vi "运维调试_氨氮.vi"() -> ()   [LabVIEW 2016, in "斯坦道氨氮.lvlib"]
uses:
  <vilib>/Utility/miscctls.llb/LVPointTypeDef.ctl
  <vilib>/Utility/config.llb/NI_LVConfig.lvlib
  <vilib>/ptbypt/NI_PtbyPt.lvlib
panel:
  out "固件版本号":string
  in  "定时设置":cluster{"启动":bool, "控制命令":T1, "测量参数":T2}(xcontrol)
  out "模块版本号":string
  in  "校准按钮":T3
  out "单位:":T4(ring)
  out "运行状态":T5 {"数据时间:" format="%<%y/%m/%d %H:%M:%S>T"; "仪器时间:" format="%<%y/%m/%d %H:%M:%S>T"}
  out "二级权限":bool
  out "一级权限":bool
  out "输入密码":u32
  out "布尔":bool
  in  "仪器参数设置":bool
  in  "流程固件":bool
  in  "量程参数读取":T6
  in  "模块启用":bool
  in  "串口设置":bool
  in  "公式一键写入":bool
  in  "流程路径":path=path "C:/Users/STD/Documents/斯坦道流程文件/流程.xml"
  in  "曲线模型":cluster{"X^2":dbl, "X":dbl, "B":dbl, "r^2":dbl}(xcontrol)
  out "字符串":string
  in  "质控参数设置":bool
  in  "自动测试量程配置":T7
  out "温度2":sgl
  out "温度1":sgl
  out "ADC":sgl
  in  "数组":string[](array[string])
  in  "量程切换阈值写入":bool
  in  "量程切换阈值读取":bool
  in  "参数下拉列表":enum16{"总磷", "总氮", "氨氮"}(ring)=enum."氨氮"
  in  "量程下拉列表":enum16{"低量程", "高量程"}(ring)
  in  "测量模式下拉列表":enum16{"水样测量", "零点核查", "跨度核查", "标样核查", "加标回收"}(ring)
  in  "公式":cluster{"X^2":dbl, "X":dbl, "b":dbl}
  in  "写公式":bool
  in  "读公式":bool
  in  "返回":bool
  in  "设置":bool
  out "集成报警信息":string
  in  "停止":bool
  in  "手动启动":bool
  in  "单步测试":bool
  out "F3":sgl format="%#.6f"
  out "F2":sgl format="%#.6f"
  out "F1":sgl format="%#.6f"
  out "F0":sgl format="%#.6f"
  out "多列列表框":i32(listbox)
  # "参数设置"
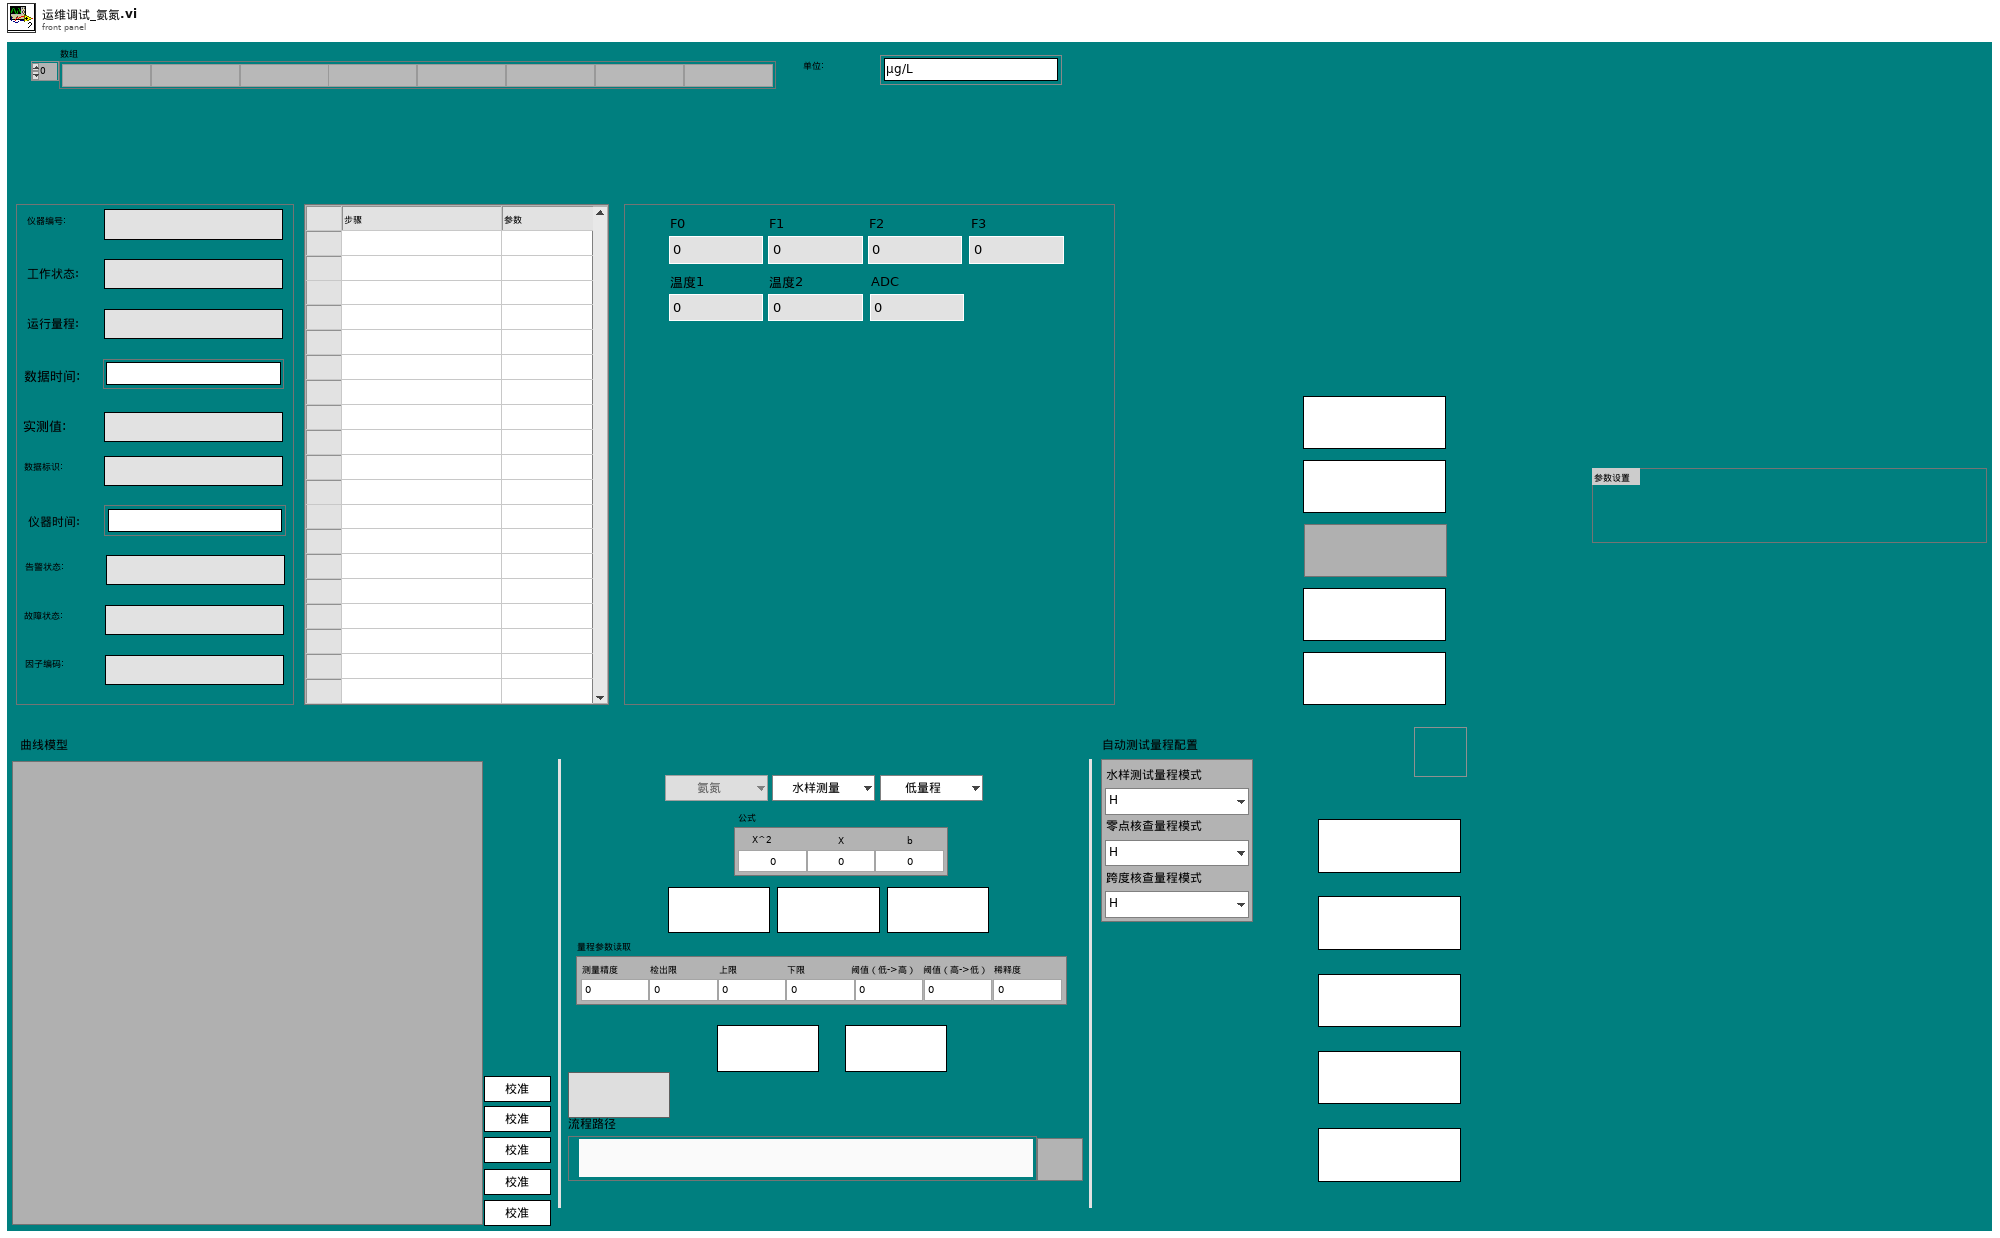
[diagram p1: front panel]
types:
  T1 = typedef "定时设置.xctl/国标控制命令.ctl" = enum16{"启动测量", "标样核查", "零点核查", "跨度核查", "空白测试", "平行样测试", "加标回收", "空白校准", "标样校准", "初始化（清洗）", "停止测试", "仪器重启", "校时", "模式设置", "测量间隔设置"}
  T2 = typedef "定时设置.xctl/测量参数.ctl" = u16
  T3 = cluster{"校准1":bool, "校准2":bool, "校准3":bool, "校准4":bool, "校准5":bool}
  T4 = enum16{"μg/L", "mg/L", "ppm", "mg/m3", "cm", "ppb", "μg/m3", "%", "nmol/mol", "μmol/mol", "MPN/L", "MPN/100ml", "ng/m3", "NTU", "无量纲", "mS/cm", "μS/cm", "℃", "mV", "cells/mL"}
  T5 = cluster{"仪器编号:":string, "工作状态:":string, "运行量程: ":string, "数据时间:":timestamp, "实测值:":string, "数据标识: ":string, "仪器时间:":timestamp, "告警状态: ":string, "故障状态:  ":string, "因子编码:":string}
  T6 = cluster{"测量精度":dbl, "检出限":dbl, "上限":dbl, "下限":dbl, "阈值（低->高）":dbl, "阈值（高->低）":dbl, "稀释度":dbl}
  T7 = cluster{"水样测试量程模式":enum16{"H", "L", "AUTO"}, "空白核查量程模式":enum16{"H", "L", "AUTO"}, "跨度核查量程模式":enum16{"H", "L", "AUTO"}}
  T8 = cluster{"时间源选择":enum16{"系统时间源", "仪器时间源"}, "外部时间源":timestamp}
  T9 = enum16{"空闲", "水样测试", "标样核查", "零点核查", "跨度核查", "空白测试", "平行样测试", "加标回收", "空白校准", "标样校准", "初始化（清洗）"}
  T10 = cluster{"系统时间":timestamp, "工作状态":enum16{"空闲", "水样测试", "标样核查", "零点核查", "跨度核查", "空白测试", "平行样测试", "加标回收", "空白校准", "标样校准", "初始化（清洗）"}, "测量模式":enum16{"待机", "连续模式", "周期模式", "定点模式", "受控模式", "手动模式"}, "告警代码":u16, "故障代码":u16, "日志代码":u16, "软件版本":u16, "F0":sgl, "F1":sgl, "F2":sgl, "F3":sgl, "T":sgl, "H":sgl, "id":u16, "flowid":u16, "量程":u16, "总磷控温温度1":sgl, "营养盐控温温度2":sgl, "ADC":sgl}
  T11 = enum32{"Bad", "Idle", "Run top level", "Running"}
  T12 = typedef "定时设置.xctl/周期模式设置.ctl" = enum16{"不启用", "定点模式", "间隔模式"}
  T13 = typedef "定时设置.xctl/定点周期设置.ctl" = cluster{"启动命令":T14, "启动命令 2":T14, "启动命令 3":T14, "启动命令 4":T14, "启动命令 5":T14, "启动命令 6":T14, "启动命令 7":T14, "启动命令 8":T14, "启动命令 9":T14, "启动命令 10":T14, "启动命令 11":T14, "启动命令 12":T14, "启动命令 13":T14, "启动命令 14":T14, "启动命令 15":T14, "启动命令 16":T14, "启动命令 17":T14, "启动命令 18":T14, "启动命令 19":T14, "启动命令 20":T14, "启动命令 21":T14, "启动命令 22":T14, "启动命令 23":T14, "启动命令 24":T14}
  T14 = typedef "定时设置.xctl/启动命令选择.ctl" = u16
  T15 = typedef "定时设置.xctl/间隔启动设置.ctl" = cluster{"启动命令":T14, "启动间隔":dbl, "启动次数":i32}
  T16 = cluster{"周期模式":T12, "定点周期":T13, "间隔启动":T15, "启动参数":u16}
  T17 = cluster{"周期模式":T12, "定点周期":T13, "间隔启动":T15, "测量参数":T2}
  T18 = typedef "LVPointTypeDef.ctl" = cluster{"Horizontal":i16, "Vertical":i16}
  T19 = cluster{"因子编码":u32, "单位":u16, "标样参考值":sgl, "水样数据时间":timestamp, "水样实测值":sgl, "水样数据标识":string, "标样数据时间":timestamp, "标样实测值":sgl, "标样数据标识":string, "空白数据时间":timestamp, "空白实测值":sgl, "空白数据标识":string, "零点核查数据时间":timestamp, "零点核查实测值":sgl, "零点核查数据标识":string, "跨度核查数据时间":timestamp, "跨度核查实测值":sgl, "跨度核查数据标识":string, "加标回收数据时间":timestamp, "加标回收实测值":sgl, "加标回收数据标识":string, "平行样数据时间":timestamp, "平行样实测值":sgl, "平行样数据标识":string, "F0":sgl, "F1":sgl, "F2":sgl, "F3":sgl, "F4":sgl, "F5":sgl, "F6":sgl, "F7":sgl, "温度":sgl, "湿度":sgl, "X值":sgl, "fidrange":u16}
  T20 = cluster{"Major":u16, "Minor":u16, "Fix":u16, "Build":u16}
  T21 = typedef "NI_LVConfig.lvlib/Config Data RefNum.ctl" = refnum<k1>
  T22 = enum8{"Enabled", "Disabled", "Disabled and Grayed Out"}
  T23 = cluster{"时间标识":timestamp, "设备":string, "日志信息":string, "备注":string}
  T24 = cluster{"参数":string, "报警内容":string, "报警分析":string}
  T25 = cluster{"启动模式":enum16{"跨度核查", "水样测量", "空白核查", "标样核查", "加标回收"}, "启动参数":u16, "量程":enum16{"低量程", "高量程"}}
  T26 = cluster{"时间标识":timestamp, "设备":string, "日志信息":string, "流程参数":string}
  T27 = typedef "LVRowAndColumnUnsignedTypeDef.ctl" = cluster{"Row":u32, "Column":u32}
  T28 = cluster{"参数下拉列表":enum16{"总磷", "总氮", "氨氮"}, "测量模式下拉列表":enum16{"水样测量", "零点核查", "跨度核查", "标样核查", "加标回收"}, "量程下拉列表":enum16{"低量程", "高量程"}}
  T29 = cluster{"站号":u16, "量程切换":enum32{"H", "L", "AUTO"}, "控制命令":enum16{"启动测量", "标样核查", "零点核查", "跨度核查", "空白测试", "平行样测试", "加标回收", "空白校准", "标样校准", "初始化（清洗）", "停止测试", "仪器重启", "校时", "模式设置", "测量间隔设置"}, "模式设置":enum16{"待机", "连续模式", "周期模式", "定点模式", "受控模式", "手动模式"}, "测量间隔":u16}
  T30 = cluster{"标液浓度1":dbl, "标液浓度2":dbl, "标液浓度3":dbl, "标液浓度4":dbl, "标液浓度5":dbl}
  T31 = cluster{"跨度值":dbl, "零点标准液浓度":dbl, "跨度标准液浓度":dbl, "标准液标准浓度":dbl}
  T32 = cluster{"确定":bool, "跨度值":dbl, "零点标准液浓度":dbl, "跨度标准液浓度":dbl, "标准液标准浓度":dbl}
  T33 = cluster{"测量量程":dbl, "测量精度":dbl, "测量间隔":dbl, "消解温度":dbl, "消解时长":dbl, "空白校准时间":timestamp, "曲线截距":dbl, "曲线斜率":dbl, "测量检出限":dbl, "测量信号值":dbl, "线性相关系数":dbl, "二次多项式系数":dbl, "标样校准时间":timestamp, "稀释倍数":dbl, "三项式系数":dbl, "空白标定系数":dbl, "量程系数":dbl, "F0/ORPA":dbl, "F1/ORPB":dbl, "F2/ORPK":dbl, "F3":dbl, "F4":dbl, "F5":dbl, "F6":dbl, "F7":dbl, "X0/滴定数":dbl, "量程":dbl}
  T34 = cluster{"确定":bool, "测量量程":dbl, "测量精度":dbl, "测量间隔":dbl, "消解温度":dbl, "消解时长":dbl, "空白校准时间":timestamp, "曲线截距":dbl, "曲线斜率":dbl, "测量检出限":dbl, "测量信号值":dbl, "线性相关系数":dbl, "二次多项式系数":dbl, "标样校准时间":timestamp, "稀释倍数":dbl, "三项式系数":dbl, "空白标定系数":dbl, "量程系数":dbl, "F0/ORPA":dbl, "F1/ORPB":dbl, "F2/ORPK":dbl, "F3":dbl, "F4":dbl, "F5":dbl, "F6":dbl, "F7":dbl, "X0/滴定数":dbl, "量程":dbl}
  T35 = cluster{"测量精度":u16, "检出限":dbl, "上限":dbl, "下限":dbl, "阈值（低->高）":dbl, "阈值（高->低）":dbl, "稀释度":dbl}
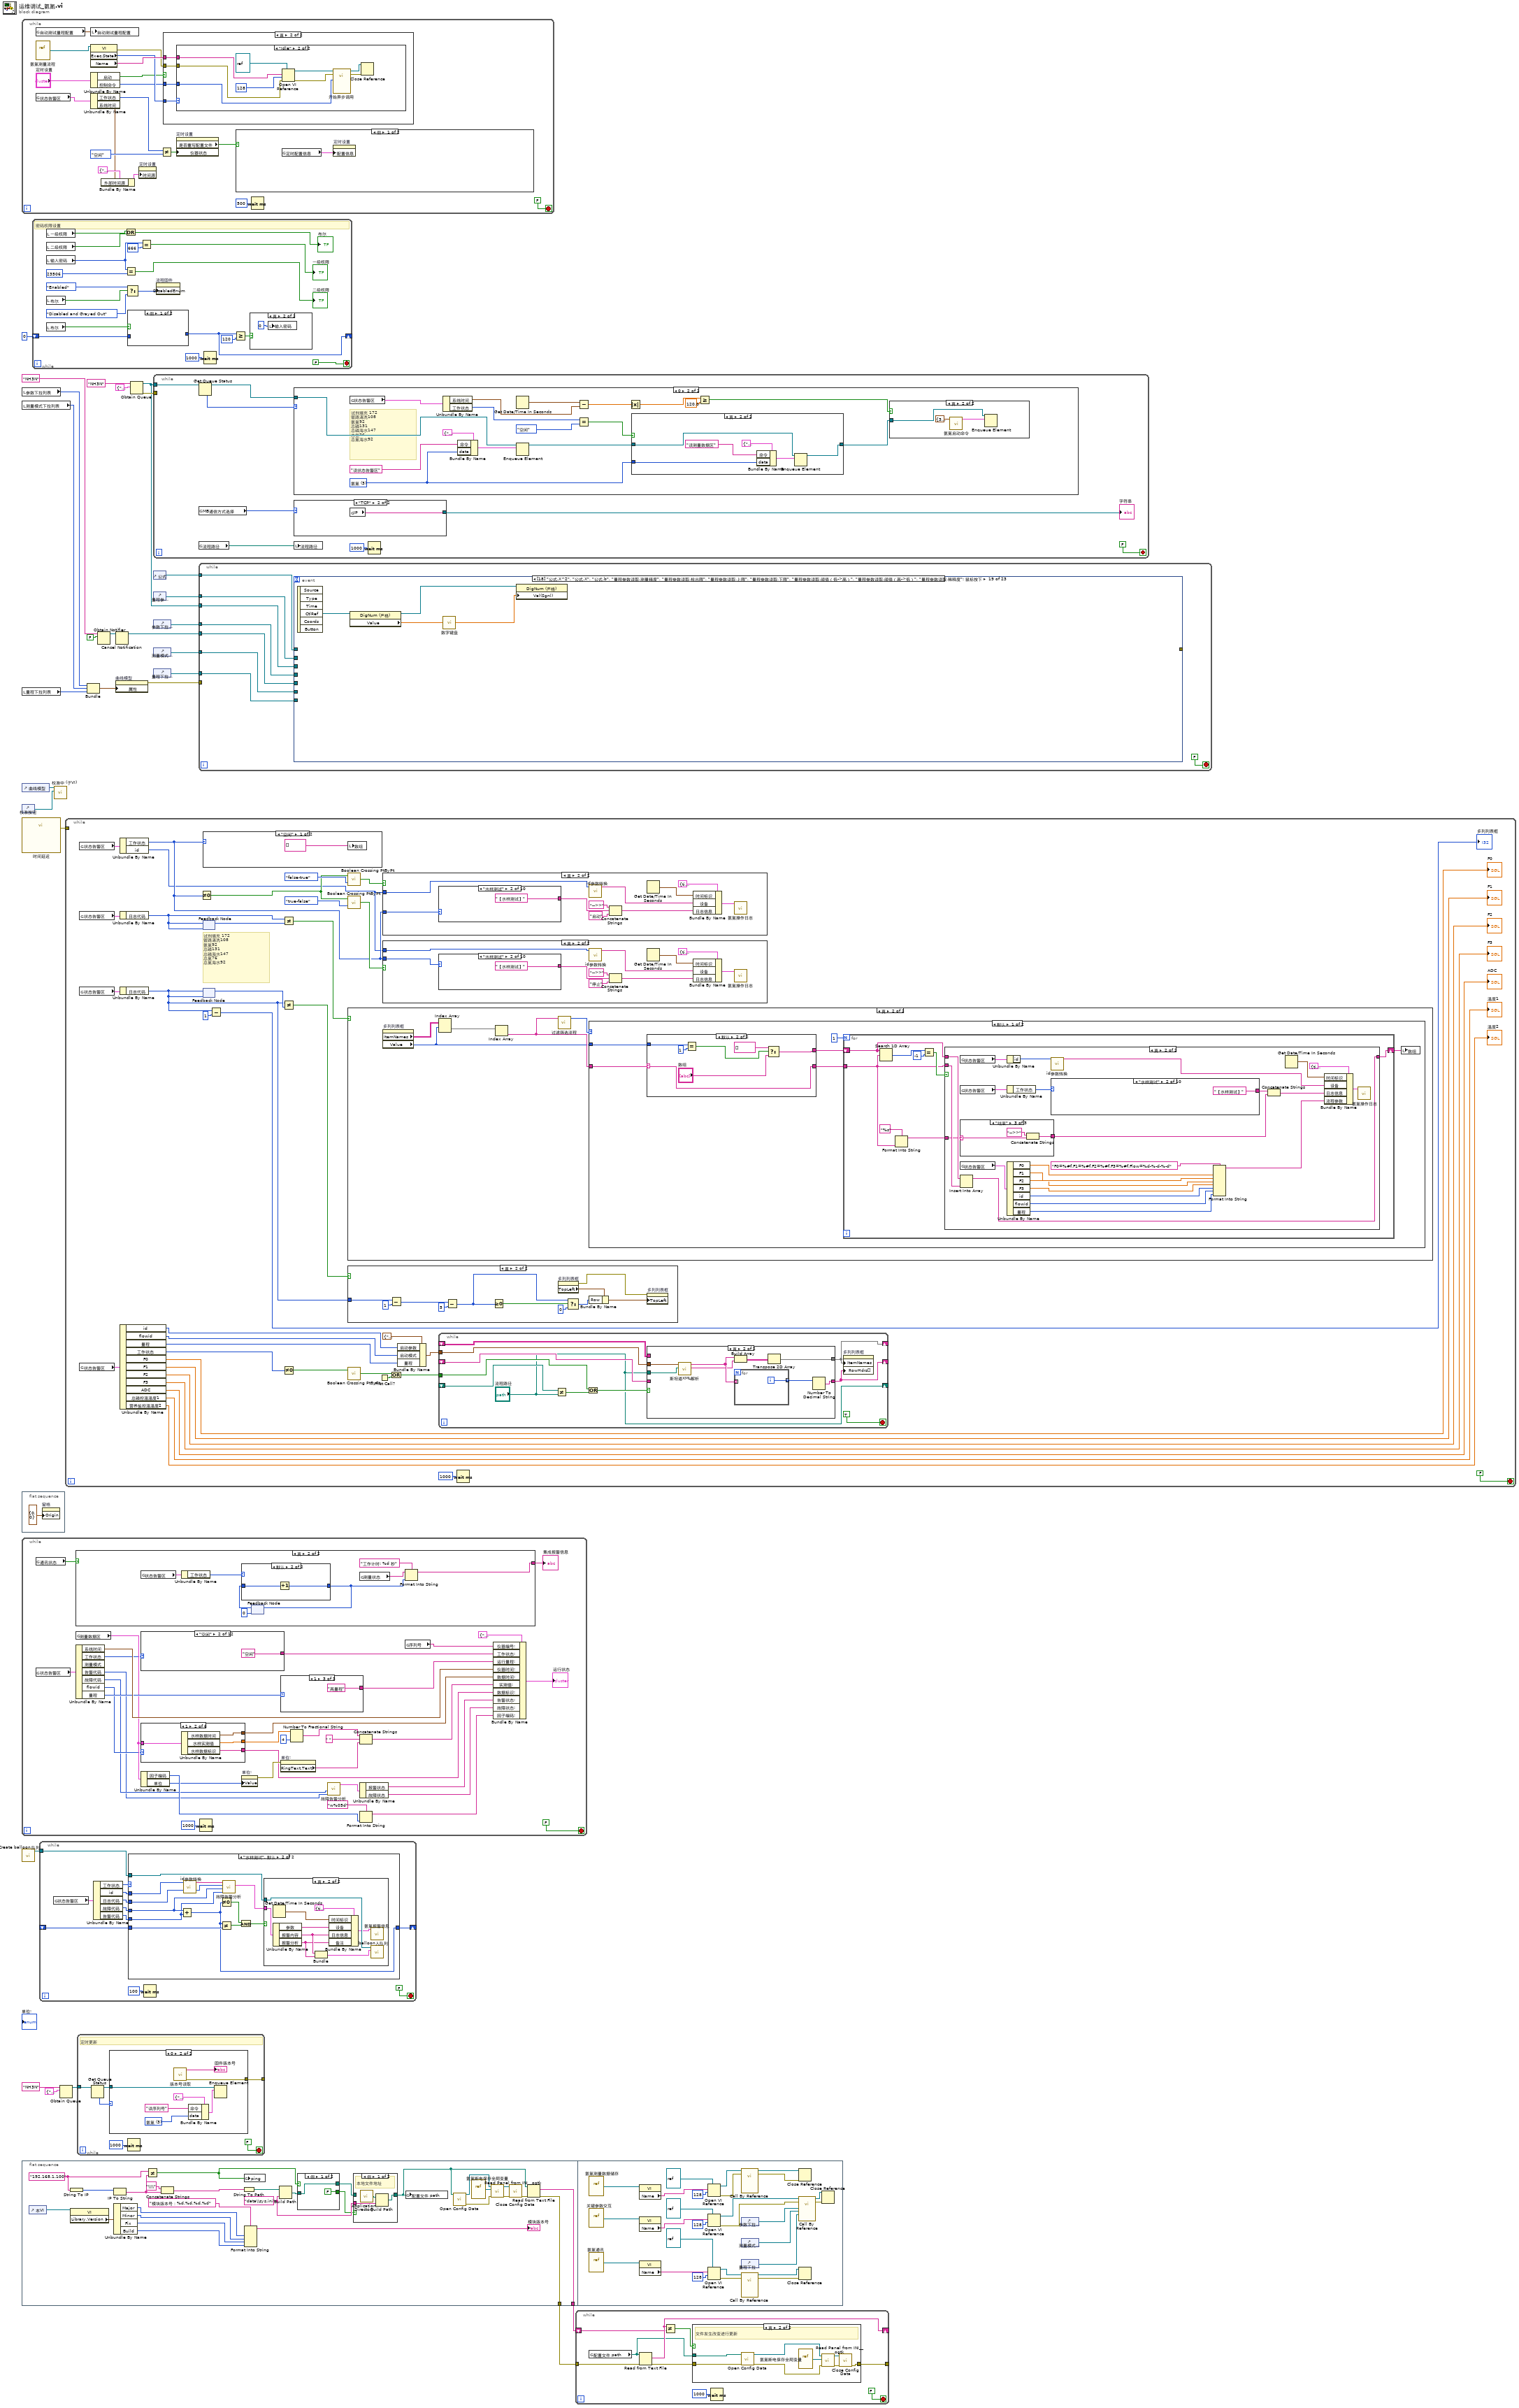
[diagram p0: block diagram]
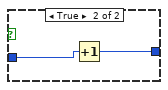
[diagram p6: hidden frame]
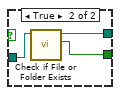
[diagram p7: hidden frame]
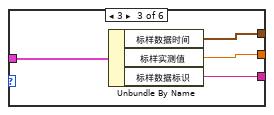
[diagram p11: hidden frame]
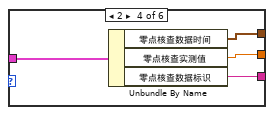
[diagram p12: hidden frame]
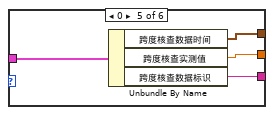
[diagram p13: hidden frame]
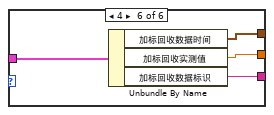
[diagram p14: hidden frame]
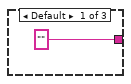
[diagram p15: hidden frame]
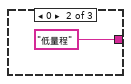
[diagram p16: hidden frame]
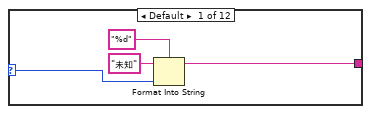
[diagram p17: hidden frame]
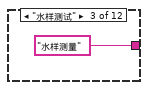
[diagram p18: hidden frame]
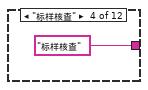
[diagram p19: hidden frame]
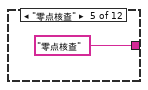
[diagram p20: hidden frame]
diagram:
  n1 = while {
    stop <- FALSE stop-if-true
    n2 = global read "氨氮断电保存全局变量.vi" "自动测试量程配置"() -> (w44:T7)
    n3 = vi-ref "氨氮测量流程.vi"() -> (w40:refnum<vi>)
    n4 = global read "VAR氨氮全局变量.vi" "状态告警区"() -> (w43:T10)
    n5 = local write "自动测试量程配置"(w44) -> ()
    n6 = property class="VI"(reference=w40) -> (error out=w37:errorcluster, "Exec.State"=w38:T11, "Name"=w39:string)  [unwired: 1 in, 1 out]
    n7 = Unbundle By Name("定时设置") -> ("启动"=w35:bool, "控制命令"=w34:T1)
    n8 = Unbundle By Name(w43) -> ("工作状态"=w42:T9, "系统时间"=w29:timestamp)
    n9 = Bundle By Name(cluster=T8 {"时间源选择"=enum."仪器时间源", "外部时间源"=timestamp(0 s since 1904-01-01)} ("时间源"), "外部时间源"=w29) -> (w30:T8)
    n10 = property on="定时设置" class="定时设置 (严格)"("时间源"=w30) -> ()  [unwired: 2 in, 2 out]
    n11 = Not Equal?(x=w42, y=T9."空闲") -> (x != y?=w32:bool)
    n12 = case shown="真" w35 {
      tunnel: w39 -> [_ w54]
      tunnel: w34 -> [_ w53]
      tunnel: w38 -> [_ w52]
      tunnel: w37 -> [_ w51]
      frame False {
      }
      frame True {
        n13 = case shown="\"Idle\"" w52 {
          tunnel: w54 -> [_ w59]
          tunnel: w53 -> [_ w57]
          tunnel: w51 -> [_ w55]
          frame "Bad", Default {
          }
          frame "Idle" {
            n14 = Open VI Reference(type specifier VI Refnum (for type only)=refnum<vi> refnum, vi path=w59, options=128 ("选项"), error in (no error)=w55) -> (vi reference=w60:refnum<vi>, error out=w61:errorcluster)  [unwired: 2 in]
            n15 = call-by-ref "开始异步调用"(reference=w60, error in=w61, "控制命令"=w57) -> (reference out=w62:refnum<vi>, error out=w63:errorcluster)  [unwired: 11 in]
            n16 = Close Reference(reference=w62, error in (no error)=w63) -> ()  [unwired: 1 out]
          }
        }
      }
    }
    n17 = property on="定时设置" class="定时设置 (严格)"("仪器状态"=w32) -> ("是否重写配置文件"=w33:bool)  [unwired: 2 in, 2 out]
    n18 = case shown="假" w33 {
      frame False {
        n19 = global read "氨氮断电保存全局变量.vi" "定时配置信息"() -> (w47:T16)
        n20 = property on="定时设置" class="定时设置 (严格)"("配置信息"=w47) -> ()  [unwired: 2 in, 2 out]
      }
      frame True {
        n21 = flat-sequence {
          tunnel: [w49] -> _
          frame #0 {
            n22 = property on="定时设置" class="定时设置 (严格)"() -> ("配置信息"=w48:T17)  [unwired: 2 in, 2 out]
            n23 = global write "氨氮断电保存全局变量.vi" "定时配置信息"(w48) -> ()
          }
          frame #1 {
            n24 = call "配置文件保存.vi"() -> ("错误输出"=w49:errorcluster)  [unwired: 11 in]
          }
          frame #2 {
            n25 = property on="定时设置" class="定时设置 (严格)"("是否重写配置文件"=FALSE) -> ()  [unwired: 2 in, 2 out]
          }
        }
      }
    }
    n26 = Wait (ms)(milliseconds to wait=u32 500 ("等待时间（毫秒）")) -> ()  [unwired: 1 out]
  }
  n27 = local read "参数下拉列表"() -> (w9:enum16{"总磷", "总氮", "氨氮"})
  n28 = local read "测量模式下拉列表"() -> (w8:enum16{"水样测量", "零点核查", "跨度核查", "标样核查", "加标回收"})
  n29 = local read "量程下拉列表"() -> (w7:enum16{"低量程", "高量程"})
  n30 = control-ref of="曲线模型"() -> (w3:refnum<vi>)
  n31 = control-ref of="校准按钮"() -> (w2:refnum<vi>)
  n32 = call "时间延迟"() -> ("error out"=w20:errorcluster)  [unwired: 11 in]
  n33 = flat-sequence {
    frame #0 {
      n34 = property on="窗格" class="Pane"("Origin"=T18 {"Horizontal"=0, "Vertical"=0} ("原点")) -> ()  [unwired: 2 in, 2 out]
    }
  }
  n35 = while {
    stop <- FALSE stop-if-true
    n36 = global read "VAR氨氮全局变量.vi" "通讯状态"() -> (w95:bool)
    n37 = global read "VAR氨氮全局变量.vi" "状态告警区"() -> (w93:T10)
    n38 = case shown="真" w95 {
      tunnel: ["通讯异常" ("集成报警信息") w138] -> w94
      frame False {
      }
      frame True {
        n39 = global read "VAR氨氮全局变量.vi" "状态告警区"() -> (w144:T10)
        n40 = Unbundle By Name(w144) -> ("工作状态"=w143:T9)
        n41 = feedback #1(0) -> (w141:i32)
        n42 = case shown="默认" w143 {
          tunnel: w141 -> [_ w146]
          tunnel: [_ w145] -> w139
          frame "空闲" {
          }
          frame Default {
            n43 = Increment(x=w146) -> (x+1=w145:i32)
          }
        }
        n44 = feedback-in #1(w139) -> ()
        n45 = global read "VAR氨氮全局变量.vi" "测量状态"() -> (w137:string)
        n46 = Format Into String(format string="工作计时: %d 秒" ("格式字符串"), initial string=w137, w139) -> (resulting string=w138:string)  [unwired: 1 in, 1 out]
      }
    }
    "集成报警信息" <- w94
    n47 = global read "VAR氨氮全局变量.vi" "测量数据区"() -> (w85:T19)
    n48 = Unbundle By Name(w93) -> ("系统时间"=w91:timestamp, "工作状态"=w84:T9, "告警代码"=w65:u16, "故障代码"=w66:u16, "flowid"=w83:u16, "量程"=w89:u16)  [unwired: 1 out]
    n49 = case shown="\"空闲\"" w84 {
      selector: w84 -> [w121 _ _ _ _ _ _ _ _ _ _ _]
      tunnel: [w122 "空闲" ("工作状态") "水样测量" ("工作状态") "标样核查" ("工作状态") "零点核查" ("工作状态") "跨度核查" ("工作状态") "空白测试" ("工作状态") "平行样测试" ("工作状态") "加标回收" ("工作状态") "空白校准" ("工作状态") "标样校准" ("工作状态") "初始化" ("工作状态")] -> w90
      frame Default {
        n50 = Format Into String(format string="%d" ("格式字符串"), initial string="未知" ("工作状态"), w121) -> (resulting string=w122:string)  [unwired: 1 in, 1 out]
      }
      frame "空闲" {
      }
      frame "水样测试" {
      }
      frame "标样核查" {
      }
      frame "零点核查" {
      }
      frame "跨度核查" {
      }
      frame "空白测试" {
      }
      frame "平行样测试" {
      }
      frame "加标回收" {
      }
      frame "空白校准" {
      }
      frame "标样校准" {
      }
      frame "初始化（清洗）" {
      }
    }
    n51 = case shown="1" w83 {
      tunnel: [_ w101 w105 w109 w113 w117] -> w74
      tunnel: [_ w99 w104 w108 w112 w116] -> w79
      tunnel: [_ w98 w103 w107 w111 w115] -> w73
      tunnel: w85 -> [_ w100 w102 w106 w110 w114]
      frame Default {
      }
      frame 1 {
        n52 = Unbundle By Name(w100) -> ("水样数据时间"=w101:timestamp, "水样实测值"=w99:sgl, "水样数据标识"=w98:string)
      }
      frame 3 {
        n53 = Unbundle By Name(w102) -> ("标样数据时间"=w105:timestamp, "标样实测值"=w104:sgl, "标样数据标识"=w103:string)
      }
      frame 2 {
        n54 = Unbundle By Name(w106) -> ("零点核查数据时间"=w109:timestamp, "零点核查实测值"=w108:sgl, "零点核查数据标识"=w107:string)
      }
      frame 0 {
        n55 = Unbundle By Name(w110) -> ("跨度核查数据时间"=w113:timestamp, "跨度核查实测值"=w112:sgl, "跨度核查数据标识"=w111:string)
      }
      frame 4 {
        n56 = Unbundle By Name(w114) -> ("加标回收数据时间"=w117:timestamp, "加标回收实测值"=w116:sgl, "加标回收数据标识"=w115:string)
      }
    }
    n57 = Unbundle By Name(w85) -> ("因子编码"=w86:u32, "单位"=w80:u16)
    n58 = Wait (ms)(milliseconds to wait=u32 1000 ("等待时间（毫秒）")) -> ()  [unwired: 1 out]
    n59 = property on="单位:" class="Enum (严格)"("Value"=w80) -> (error out=w81:errorcluster)  [unwired: 2 in, 1 out]
    n60 = case shown="1" w89 {
      tunnel: ["" ("字符串") "低量程" ("字符串") "高量程" ("字符串")] -> w88
      frame Default {
      }
      frame 0 {
      }
      frame 1 {
      }
    }
    n61 = property on="单位:" class="Enum (严格)"(error in=w81) -> ("RingText.Text"=w70:string)  [unwired: 1 in, 2 out]
    n62 = Number To Fractional String(number=w79, precision (6)=i16 4 ("精度(6)")) -> (F-format string=w77:string)  [unwired: 2 in]
    n63 = call "故障告警分析.vi"("告警代码"=w65, "故障代码"=w66) -> ("简易报警状态"=w69:cluster{"故障状态":string, "报警状态":string})  [unwired: 8 in, 1 out]
    n64 = Concatenate Strings(w77, " " ("字符串"), w70) -> (w76:string)
    n65 = Unbundle By Name(w69) -> ("报警状态"=w68:string, "故障状态"=w67:string)
    n66 = Format Into String(format string="w%05d" ("格式字符串"), w86) -> (resulting string=w75:string)  [unwired: 2 in, 1 out]
    n67 = global read "VAR氨氮全局变量.vi" "序列号"() -> (w92:string)
    n68 = Bundle By Name(cluster=T5 {"仪器编号:"="", "工作状态:"="", "运行量程: "="", "数据时间:"=timestamp(0 s since 1904-01-01), "实测值:"="", "数据标识: "="", "仪器时间:"=timestamp(0 s since 1904-01-01), "告警状态: "="", "故障状态:  "="", "因子编码:"=""} ("运行状态"), "仪器编号:"=w92, "工作状态:"=w90, "运行量程:"=w88, "仪器时间:"=w91, "数据时间:"=w74, "实测值:"=w76, "数据标识:"=w73, "告警状态:"=w68, "故障状态:"=w67, "因子编码:"=w75) -> (→"运行状态":T5)
  }
  n69 = call "Create balloon 队列.vi"() -> ("队列输出"=w1:refnum<queue>)  [unwired: 11 in]
  n70 = flat-sequence {
    tunnel: [w156] -> w5
    tunnel: [w155] -> w4
    frame #0 {
      w168 = "data\\sys.ini" ("名称或相对路径")
      w160 = "192.168.1.100" ("名称")
      n71 = control-ref of="本VI"() -> (w154:refnum<vi>)
      n72 = String To IP(1:w160) -> (0:w167:u32)
      n73 = property class="VI"(reference=w154) -> ("Library.Version"=w153:T20)  [unwired: 1 in, 2 out]
      n74 = IP To String(2:w167) -> (0:w164:string)  [unwired: 1 in]
      n75 = Unbundle By Name(w153) -> ("Major"=w151:u16, "Minor"=w150:u16, "Fix"=w149:u16, "Build"=w148:u16)
      n76 = Not Equal?(x=w160, y=w164) -> (x != y?=w169:bool)
      n77 = Concatenate Strings("\\\\" ("字符串"), w164) -> (w165:string)
      n78 = String To Path(string=w165) -> (path=w159:path)
      n79 = global write "VAR氨氮全局变量.vi" "ping"(w169) -> ()
      n80 = Format Into String(format string="模块版本号：%d.%d.%d.%d" ("格式字符串"), w151, w150, w149, w148) -> (resulting string=→"模块版本号":string)  [unwired: 2 in, 1 out]
      n81 = Build Path(base path=w159, name or relative path=w168) -> (appended path=w163:path)
      n82 = case shown="假" w169 {
        tunnel: w163 -> [w175 w179]
        tunnel: [w175 w178] -> w162
        tunnel: [FALSE w177] -> w161
        frame False {
        }
        frame True {
          n83 = call <vilib>:"Check if File or Folder Exists.vi"("path"=w179) -> ("file or folder exists?"=w177:bool, "dup path"=w178:path)  [unwired: 8 in, 1 out]
        }
      }
      n84 = case shown="假" w161 {
        tunnel: w162 -> [_ w183]
        tunnel: [w181 w183] -> w158
        tunnel: w168 -> [w180 _]
        frame False {
          # "本地文件地址"
          n85 = call <vilib>:"Application Directory.vi"() -> ("Application Directory"=w182:path)
          n86 = Build Path(base path=w182, name or relative path=w180) -> (appended path=w181:path)
        }
        frame True {
          # "网络共享地址"
        }
      }
      n87 = global write "VAR氨氮全局变量.vi" "配置文件 path"(w158) -> ()
      n88 = call <vilib>:"Open Config Data.vi"("configuration file path"=w158) -> ("error out"=w171:errorcluster, "refnum"=w174:T21)  [unwired: 8 in, 1 out]
      n89 = vi-ref "氨氮断电保存全局变量.vi"() -> (w173:refnum<vi>)
      n90 = call <userlib>:"Read Panel from INI__ogtk.vi"("error in (no error)"=w171, "VI ref"=w173, "refnum"=w174) -> ("error out"=w170:errorcluster, "refnum out"=w172:T21)  [unwired: 7 in]
      n91 = call <vilib>:"Close Config Data.vi"("error in (no error)"=w170, "refnum"=w172) -> ("error out"=w157:errorcluster)  [unwired: 8 in, 1 out]
      n92 = Read from Text File(file (use dialog)=w158, error in=w157) -> (text=w155:string, error out=w156:errorcluster)  [unwired: 2 in, 2 out]
    }
    frame #1 {
      n93 = vi-ref "氨氮测量数据储存.vi"() -> (w202:refnum<vi>)
      n94 = vi-ref "关键参数交互.vi"() -> (w187:refnum<vi>)
      n95 = vi-ref "氨氮通讯.vi"() -> (w210:refnum<vi>)
      n96 = property class="VI"(reference=w202) -> ("Name"=w195:string)  [unwired: 1 in, 2 out]
      n97 = property class="VI"(reference=w187) -> ("Name"=w194:string)  [unwired: 1 in, 2 out]
      n98 = property class="VI"(reference=w210) -> ("Name"=w209:string)  [unwired: 1 in, 2 out]
      n99 = Open VI Reference(type specifier VI Refnum (for type only)=refnum<vi> refnum, vi path=w195, options=128 ("选项")) -> (vi reference=w197:refnum<vi>, error out=w199:errorcluster)  [unwired: 3 in]
      n100 = Open VI Reference(type specifier VI Refnum (for type only)=refnum<vi> refnum, vi path=w194, options=128 ("选项")) -> (vi reference=w192:refnum<vi>, error out=w190:errorcluster)  [unwired: 3 in]
      n101 = Open VI Reference(type specifier VI Refnum (for type only)=refnum<vi> refnum, vi path=w209, options=128 ("选项")) -> (vi reference=w207:refnum<vi>, error out=w205:errorcluster)  [unwired: 3 in]
      n102 = call-by-ref "?"(reference=w197, error in=w199) -> (reference out=w201:refnum<vi>, error out=w200:errorcluster)  [unwired: 12 in]
      n103 = control-ref of="参数下拉列表"() -> (w186:refnum<vi>)
      n104 = control-ref of="测量模式下拉列表"() -> (w185:refnum<vi>)
      n105 = control-ref of="量程下拉列表"() -> (w184:refnum<vi>)
      n106 = call-by-ref "?"(reference=w207, error in=w205) -> (reference out=w203:refnum<vi>, error out=w204:errorcluster)  [unwired: 12 in]
      n107 = Close Reference(reference=w201, error in (no error)=w200) -> ()  [unwired: 1 out]
      n108 = call-by-ref "?"(reference=w192, error in=w190, "量程下拉列表"=w184, "测量模式下拉列表"=w185, "参数下拉列表"=w186) -> (reference out=w188:refnum<vi>, error out=w189:errorcluster)  [unwired: 9 in]
      n109 = Close Reference(reference=w203, error in (no error)=w204) -> ()  [unwired: 1 out]
      n110 = Close Reference(reference=w188, error in (no error)=w189) -> ()  [unwired: 1 out]
    }
  }
  n111 = while {
    shift-right: [w213] -> _
    shift-left: u32 0 ("等待时间（毫秒）") -> [w214]
    stop <- FALSE stop-if-true
    # "密码权限设置"
    n112 = local read "一级权限"() -> (w222:bool)
    n113 = local read "二级权限"() -> (w223:bool)
    n114 = local read "输入密码"() -> (w226:u32)
    n115 = local read "布尔"() -> (w217:bool)
    n116 = local read "布尔"() -> (w215:bool)
    n117 = Or(x=w222, y=w223) -> (x .or. y?=→"布尔":bool)
    n118 = Equal?(x=w226, y=u32 23506) -> (x = y?=→"二级权限":bool)
    n119 = Select(t=T22."Enabled" ("禁用"), s=w217, f=T22."Disabled and Grayed Out") -> (s? t:f=w218:T22)
    n120 = case shown="假" w215 {
      tunnel: w214 -> [_ w232]
      tunnel: [_ w231] -> w213
      frame False {
      }
      frame True {
        n121 = Increment(x=w232) -> (x+1=w231:u32)
      }
    }
    n122 = Equal?(x=w226, y=u32 666) -> (x = y?=→"一级权限":bool)
    n123 = property on="流程固件" class="Bool"("DisabledEnum"=w218) -> ()  [unwired: 2 in, 2 out]
    n124 = Wait (ms)(milliseconds to wait=u32 1000 ("等待时间（毫秒）")) -> ()  [unwired: 1 out]
    n125 = Greater Or Equal?(x=w213, y=u32 120) -> (x >= y?=w211:bool)
    n126 = case shown="真" w211 {
      frame False {
      }
      frame True {
        n127 = local write "输入密码"(u32 0 ("输入密码")) -> ()
      }
    }
  }
  n128 = while {
    tunnel: w1 -> [w238]
    shift-right: [w234] -> _
    shift-left: _ -> [w235]
    stop <- FALSE stop-if-true
    n129 = global read "VAR氨氮全局变量.vi" "状态告警区"() -> (w242:T10)
    n130 = Unbundle By Name(w242) -> ("工作状态"=w233:T9, "id"=w240:u16, "日志代码"=w239:u16, "故障代码"=w237:u16, "告警代码"=w236:u16)
    n131 = case shown="\"水样测试\", 默认" w233 {
      tunnel: w240 -> [_ w256]
      tunnel: w239 -> [_ w255]
      tunnel: w238 -> [_ w252]
      tunnel: w237 -> [_ w251]
      tunnel: w236 -> [_ w250]
      tunnel: w235 -> [w244 w249]
      tunnel: [w244 w248] -> w234
      frame "空闲" {
      }
      frame "水样测试", Default {
        n132 = Add(x=w251, y=w250) -> (x+y=w248:u16)
        n133 = call "id参数转换.vi"("id"=w256) -> ("table输出"=w253:string)  [unwired: 10 in]
        n134 = Not Equal To 0?(x=w248) -> (x != 0?=w247:bool)
        n135 = Not Equal?(x=w248, y=w249) -> (x != y?=w246:bool)
        n136 = call "故障告警分析.vi"("告警代码"=w250, "故障代码"=w251, "运行步序"=w255, "参数"=w253) -> ("报警内容"=w254:T24)  [unwired: 6 in, 1 out]
        n137 = And(x=w247, y=w246) -> (x .and. y?=w245:bool)
        n138 = case shown="真" w245 {
          tunnel: w254 -> [_ w265]
          tunnel: w252 -> [_ w264]
          frame False {
          }
          frame True {
            n139 = Get Date/Time In Seconds() -> (seconds since 1Jan1904=w263:timestamp)
            n140 = Unbundle By Name(w265) -> ("参数"=w260:string, "报警内容"=w259:string, "报警分析"=w258:string)
            n141 = Bundle("报警内容"=w259, "报警分析"=w258) -> (w257:cluster{"报警内容":string, "报警分析":string})  [unwired: 1 in]
            n142 = Bundle By Name(cluster=T23 {"时间标识"=timestamp(0 s since 1904-01-01), "设备"="", "日志信息"="", "备注"=""} ("data in"), "时间标识"=w263, "设备"=w260, "日志信息"=w259, "备注"=w258) -> (w262:T23)
            n143 = call "氨氮报警信息.vi"("data in"=w262) -> ()  [unwired: 10 in, 1 out]
            n144 = call "balloon入队列.vi"("报警内容"=w257, "队列"=w264) -> ()  [unwired: 9 in, 1 out]
          }
        }
      }
    }
    n145 = Wait (ms)(milliseconds to wait=u32 100) -> ()  [unwired: 1 out]
  }
  n146 = call "校准中 (子VI).vi"("曲线模型"=w3, "校准按钮"=w2) -> ()  [unwired: 9 in]
  n147 = Obtain Queue(name (unnamed)="NH3N" ("名称（未命名）"), element data type=cluster{"命令":string, "data":variant} {"命令"="", "data"=variant}) -> (queue out=w17:refnum<queue>)  [unwired: 3 in, 2 out]
  n148 = while {
    tunnel: w20 -> [_]
    stop <- FALSE stop-if-true
    # "试剂填充 172 \n管路清洗108\n氨氮92\n总磷131\n总磷海水147\n总氮76\n总氮海水92"
    n149 = global read "VAR氨氮全局变量.vi" "状态告警区"() -> (w286:T10)
    n150 = global read "VAR氨氮全局变量.vi" "状态告警区"() -> (w284:T10)
    n151 = global read "VAR氨氮全局变量.vi" "状态告警区"() -> (w288:T10)
    n152 = global read "VAR氨氮全局变量.vi" "状态告警区"() -> (w296:T10)
    n153 = Unbundle By Name(w286) -> ("工作状态"=w267:T9, "id"=w266:u16)
    n154 = Unbundle By Name(w284) -> ("日志代码"=w283:u16)
    n155 = Unbundle By Name(w288) -> ("日志代码"=w280:u16)
    n156 = Unbundle By Name(w296) -> ("id"=w293:u16, "flowid"=w295:u16, "量程"=w294:u16, "工作状态"=w274:T9, "F0"=→"F0":sgl, "F1"=→"F1":sgl, "F2"=→"F2":sgl, "F3"=→"F3":sgl, "ADC"=→"ADC":sgl, "总磷控温温度1"=→"温度1":sgl, "营养盐控温温度2"=→"温度2":sgl)
    n157 = Not Equal To 0?(x=w267) -> (x != 0?=w269:bool)
    n158 = case shown="\"空闲\"" w267 {
      frame "空闲" {
        n159 = local write "数组"(string[] [] ("数组")) -> ()
      }
      frame "水样测试", Default {
      }
    }
    n160 = feedback #2(w283) -> (w285:u16)
    n161 = feedback-in #2(w283) -> ()
    n162 = feedback-in #3(w280) -> ()
    n163 = feedback #3(w280) -> (w301:u16)
    n164 = Subtract(x=w280, y=1) -> (x-y=→"多列列表框":i32)
    n165 = Not Equal?(x=w283, y=w285) -> (x != y?=w282:bool)
    n166 = Not Equal?(x=w280, y=w301) -> (x != y?=w300:bool)
    n167 = Not Equal To 0?(x=w274) -> (x != 0?=w298:bool)
    n168 = call <vilib>:"Boolean Crossing PtByPt.vi"("direction"=enum16{"either", "false-true", "true-false"}."false-true", "input"=w269) -> ("crossing"=w271:bool)  [unwired: 1 in]
    n169 = call <vilib>:"Boolean Crossing PtByPt.vi"("direction"=enum16{"either", "false-true", "true-false"}."true-false", "input"=w269) -> ("crossing"=w268:bool)  [unwired: 1 in]
    n170 = case shown="真" w282 {
      frame False {
      }
      frame True {
        n171 = property on="多列列表框" class="MCListbox (严格)"() -> ("ItemNames"=w347:string[][], "Value"=w343:i32)  [unwired: 2 in, 2 out]
        n172 = Index Array(array=w347, index (row)=w343) -> (element=w346:string[])  [unwired: 1 in]
        n173 = Index Array(array=w346) -> (element=w345:string)  [unwired: 1 in]
        n174 = call "过滤筛选流程.vi"("字符串"=w345) -> ("匹配后偏移量"=w344:i32)  [unwired: 10 in]
        n175 = case shown="默认" w344 {
          tunnel: w345 -> [w349 _]
          tunnel: w343 -> [w348 _]
          frame Default {
            n176 = case shown="默认" w349 {
              selector: w349 -> [w355 w362]
              tunnel: [w355 w362] -> w351
              tunnel: [string[] [] ("数组") w357] -> w350
              tunnel: w348 -> [_ w361]
              frame "读数" {
              }
              frame Default {
                n177 = Equal?(x=w361, y=1) -> (x = y?=w359:bool)
                n178 = Select(t=string[] [], s=w359, f="数组") -> (s? t:f=w357:string[])
              }
            }
            n179 = for {
              N: 1 -> [_]
              tunnel: w351 -> [w364]
              shift-right: [w363] -> w352
              shift-left: w350 -> [w365]
              n180 = Search 1D Array(1D array=w365, element=w364) -> (index of element=w368:i32)  [unwired: 1 in]
              n181 = Format Into String(format string="%s" ("格式字符串"), w364) -> (resulting string=w369:string)  [unwired: 2 in, 1 out]
              n182 = Equal?(x=w368, y=-1) -> (x = y?=w366:bool)
              n183 = case shown="真" w366 {
                tunnel: w369 -> [_ w379]
                tunnel: w365 -> [w371 w383]
                tunnel: w364 -> [_ w382]
                tunnel: [w371 w381] -> w363
                frame False {
                }
                frame True {
                  n184 = global read "VAR氨氮全局变量.vi" "状态告警区"() -> (w396:T10)
                  n185 = global read "VAR氨氮全局变量.vi" "状态告警区"() -> (w378:T10)
                  n186 = case shown="\"结束\"" w379 {
                    selector: w379 -> [w406 w409 w412]
                    tunnel: [w406 w408 w411] -> w375
                    frame Default {
                    }
                    frame "初始化" {
                      n187 = Concatenate Strings("-->>" ("字符串"), w409) -> (w408:string)
                    }
                    frame "结束" {
                      n188 = Concatenate Strings("-->>" ("字符串"), w412) -> (w411:string)
                    }
                  }
                  n189 = global read "VAR氨氮全局变量.vi" "状态告警区"() -> (w393:T10)
                  n190 = Insert Into Array(array=w383, new element=w382) -> (w381:string[])  [unwired: 1 in]
                  n191 = Unbundle By Name(w396) -> ("id"=w373:u16)
                  n192 = Unbundle By Name(w378) -> ("工作状态"=w377:T9)
                  n193 = Unbundle By Name(w393) -> ("F0"=w390:sgl, "F1"=w389:sgl, "F2"=w388:sgl, "F3"=w387:sgl, "id"=w386:u16, "flowid"=w385:u16, "量程"=w384:u16)
                  n194 = call "id参数转换.vi"("id"=w373) -> ("table输出"=w372:string)  [unwired: 10 in]
                  n195 = case shown="\"水样测试\"" w377 {
                    tunnel: [_ "【水样测试】" ("字符串") "【标样核查】" ("字符串") "【零点核查】" ("字符串") "【跨度核查】" ("字符串") "【空白测试】" ("字符串") "【平行样测试】" ("字符串") "【加标回收】" ("字符串") "【空白校准】" ("字符串") "【标样校准】" ("字符串")] -> w376
                    frame "空闲", Default {
                    }
                    frame "水样测试" {
                    }
                    frame "标样核查" {
                    }
                    frame "零点核查" {
                    }
                    frame "跨度核查" {
                    }
                    frame "空白测试" {
                    }
                    frame "平行样测试" {
                    }
                    frame "加标回收" {
                    }
                    frame "空白校准" {
                    }
                    frame "标样校准" {
                    }
                  }
                  n196 = Format Into String(format string="F0=%#f,F1=%#f,F2=%#f,F3=%#f,Flow=%d-%-d-%-d" ("格式字符串"), w390, w389, w388, w387, w386, w385, w384) -> (resulting string=w391:string)  [unwired: 2 in, 1 out]
                  n197 = Concatenate Strings(w376, w375) -> (w374:string)
                  n198 = Get Date/Time In Seconds() -> (seconds since 1Jan1904=w394:timestamp)
                  n199 = Bundle By Name(cluster=T26 {"时间标识"=timestamp(0 s since 1904-01-01), "设备"="", "日志信息"="", "流程参数"=""} ("data in"), "时间标识"=w394, "设备"=w372, "日志信息"=w374, "流程参数"=w391) -> (w395:T26)
                  n200 = call "氨氮操作日志.vi"("data in"=w395) -> ()  [unwired: 11 in]
                }
              }
            }
            n201 = local write "数组"(w352) -> ()
          }
          frame -1 {
          }
        }
      }
    }
    n202 = case shown="真" w300 {
      tunnel: w280 -> [_ w437]
      frame False {
      }
      frame True {
        n203 = Subtract(x=w437, y=1) -> (x-y=w435:i32)
        n204 = Subtract(x=w435, y=5) -> (x-y=w439:i32)
        n205 = Greater Or Equal To 0?(x=w439) -> (x >= 0?=w438:bool)
        n206 = property on="多列列表框" class="MCListbox (严格)"() -> (error out=w443:errorcluster, "TopLeft"=w444:T27)  [unwired: 2 in, 1 out]
        n207 = Select(t=w439, s=w438, f=0) -> (s? t:f=w440:i32)
        n208 = Bundle By Name(cluster=w444, "Row"=w440) -> (w445:T27)
        n209 = property on="多列列表框" class="MCListbox (严格)"(error in=w443, "TopLeft"=w445) -> ()  [unwired: 1 in, 2 out]
      }
    }
    n210 = call <vilib>:"Boolean Crossing PtByPt.vi"("input"=w298) -> ("crossing"=w273:bool)  [unwired: 2 in]
    n211 = First Call?() -> (First Call?: T/F=w299:bool)
    n212 = case shown="真" w271 {
      tunnel: w266 -> [_ w324]
      tunnel: w267 -> [_ w329]
      frame False {
      }
      frame True {
        n213 = case shown="\"水样测试\"" w329 {
          tunnel: [_ "【水样测试】" ("字符串") "【标样核查】" ("字符串") "【零点核查】" ("字符串") "【跨度核查】" ("字符串") "【空白测试】" ("字符串") "【平行样测试】" ("字符串") "【加标回收】" ("字符串") "【空白校准】" ("字符串") "【标样校准】" ("字符串")] -> w328
          frame "空闲", Default {
          }
          frame "水样测试" {
          }
          frame "标样核查" {
          }
          frame "零点核查" {
          }
          frame "跨度核查" {
          }
          frame "空白测试" {
          }
          frame "平行样测试" {
          }
          frame "加标回收" {
          }
          frame "空白校准" {
          }
          frame "标样校准" {
          }
        }
        n214 = call "id参数转换.vi"("id"=w324) -> ("table输出"=w323:string)  [unwired: 10 in]
        n215 = Concatenate Strings("-->>" ("字符串"), w328, "启动" ("字符串")) -> (w327:string)
        n216 = Get Date/Time In Seconds() -> (seconds since 1Jan1904=w331:timestamp)
        n217 = Bundle By Name(cluster=T26 {"时间标识"=timestamp(0 s since 1904-01-01), "设备"="", "日志信息"="", "流程参数"=""} ("data in"), "时间标识"=w331, "设备"=w323, "日志信息"=w327) -> (w330:T26)
        n218 = call "氨氮操作日志.vi"("data in"=w330) -> ()  [unwired: 11 in]
      }
    }
    n219 = case shown="真" w268 {
      tunnel: w266 -> [_ w305]
      tunnel: w267 -> [_ w310]
      frame False {
      }
      frame True {
        n220 = case shown="\"水样测试\"" w310 {
          tunnel: [_ "【水样测试】" ("字符串") "【标样核查】" ("字符串") "【零点核查】" ("字符串") "【跨度核查】" ("字符串") "【空白测试】" ("字符串") "【平行样测试】" ("字符串") "【加标回收】" ("字符串") "【空白校准】" ("字符串") "【标样校准】" ("字符串")] -> w309
          frame "空闲", Default {
          }
          frame "水样测试" {
          }
          frame "标样核查" {
          }
          frame "零点核查" {
          }
          frame "跨度核查" {
          }
          frame "空白测试" {
          }
          frame "平行样测试" {
          }
          frame "加标回收" {
          }
          frame "空白校准" {
          }
          frame "标样校准" {
          }
        }
        n221 = call "id参数转换.vi"("id"=w305) -> ("table输出"=w304:string)  [unwired: 10 in]
        n222 = Concatenate Strings("-->>" ("字符串"), w309, "停止" ("字符串")) -> (w308:string)
        n223 = Get Date/Time In Seconds() -> (seconds since 1Jan1904=w312:timestamp)
        n224 = Bundle By Name(cluster=T26 {"时间标识"=timestamp(0 s since 1904-01-01), "设备"="", "日志信息"="", "流程参数"=""} ("data in"), "时间标识"=w312, "设备"=w304, "日志信息"=w308) -> (w311:T26)
        n225 = call "氨氮操作日志.vi"("data in"=w311) -> ()  [unwired: 11 in]
      }
    }
    n226 = Or(x=w273, y=w299) -> (x .or. y?=w297:bool)
    n227 = Bundle By Name(cluster=T25 {"启动模式"=enum."跨度核查", "启动参数"=1, "量程"=enum."低量程"} ("参数簇"), "启动参数"=w293, "启动模式"=w295, "量程"=w294) -> (w287:T25)
    n228 = while {
      tunnel: w297 -> [w423]
      tunnel: w287 -> [w422]
      shift-right: [w417] -> _
      shift-left: _ -> [w419]
      shift-right: [w418] -> _
      shift-left: _ -> [w420]
      shift-right: ["流程路径"] -> _
      shift-left: _ -> [w416]
      stop <- TRUE stop-if-true
      n229 = Not Equal?(x=w416, y="流程路径") -> (x != y?=w414:bool)
      n230 = Or(x=w423, y=w414) -> (x .or. y?=w415:bool)
      n231 = case shown="真" w415 {
        tunnel: [w425 w433] -> w418
        tunnel: [w424 w432] -> w417
        tunnel: w422 -> [_ w427]
        tunnel: w420 -> [w425 _]
        tunnel: w419 -> [w424 _]
        tunnel: "流程路径" -> [_ w426]
        frame False {
        }
        frame True {
          n232 = call "斯坦道XML解析.vi"("添加的路径"=w426, "参数簇"=w427) -> ("步骤时间"=w428:string[], "步骤名"=w430:string[])  [unwired: 8 in]
          n233 = Build Array(w430, w428) -> (w429:string[][])
          n234 = for {
            tunnel: w430 -> [_] mode=indexing
            tunnel: [w434] -> w431 mode=indexing
            i -> [w434]
          }
          n235 = Transpose 2D Array(2D array=w429) -> (transposed array=w432:string[][])
          n236 = Number To Decimal String(number=w431) -> (decimal integer string=w433:string[])  [unwired: 1 in]
        }
      }
      n237 = property on="多列列表框" class="MCListbox (严格)"("ItemNames"=w417, "RowHdrs[]"=w418) -> ()  [unwired: 2 in, 2 out]
    }
    n238 = Wait (ms)(milliseconds to wait=u32 1000 ("等待时间（毫秒）")) -> ()  [unwired: 1 out]
  }
  n239 = while {
    tunnel: w17 -> [w450]
    tunnel: [w448] -> _
    stop <- FALSE stop-if-true
    # "定时更新"
    n240 = Get Queue Status(queue=w450) -> (queue out=w447:refnum<queue>, # elements in queue=w446:i32)  [unwired: 2 in, 6 out]
    n241 = case shown="0" w446 {
      tunnel: [_ w454] -> w448
      tunnel: w447 -> [_ w453]
      frame Default {
      }
      frame 0 {
        w456 = u16 3 items=["总磷"=1, "氨氮"=3] ("站号")
        n242 = call "版本号读取.vi"() -> ("error out"=w454:errorcluster, "固件版本号"=→"固件版本号":string)  [unwired: 10 in]
        n243 = Bundle By Name(cluster=cluster{"命令":string, "data":variant} {"命令"="", "data"=variant} ("元素"), "命令"="读序列号", "data"=w456) -> (w455:cluster{"命令":string, "data":variant})
        n244 = Enqueue Element(queue=w453, element=w455) -> ()  [unwired: 2 in, 3 out]
      }
    }
    n245 = Wait (ms)(milliseconds to wait=u32 1000 ("等待时间（毫秒）")) -> ()  [unwired: 1 out]
  }
  n246 = Bundle("参数下拉列表"=w9, "测量模式下拉列表"=w8, "量程下拉列表"=w7) -> (w10:T28)  [unwired: 1 in]
  n247 = Obtain Notifier(name (unnamed)="NH3N" ("名称（未命名）"), notification data type=FALSE) -> (notifier out=w13:refnum<notifier>)  [unwired: 2 in, 2 out]
  n248 = Cancel Notification(0:w13) -> (8:w12:refnum<notifier>)  [unwired: 1 in, 2 out]
  n249 = property on="曲线模型" class="曲线模型 (严格)"("属性"=w10) -> (error out=w16:errorcluster)  [unwired: 2 in, 1 out]
  n250 = Obtain Queue(name (unnamed)="NH3N" ("名称（未命名）"), element data type=cluster{"命令":string, "data":variant} {"命令"="", "data"=variant}) -> (queue out=w25:refnum<queue>, error out=w26:errorcluster)  [unwired: 3 in, 1 out]
  n251 = while {
    tunnel: w25 -> [w464]
    tunnel: w26 -> [_]
    stop <- FALSE stop-if-true
    n252 = Get Queue Status(queue=w464) -> (queue out=w460:refnum<queue>, # elements in queue=w459:i32)  [unwired: 2 in, 6 out]
    n253 = global read "氨氮断电保存全局变量.vi" "MB通信方式选择"() -> (w461:enum16{"串口", "TCP"})
    n254 = global read "氨氮断电保存全局变量.vi" "流程路径"() -> (w463:path)
    n255 = case shown="0" w459 {
      tunnel: w460 -> [_ w470]
      frame Default {
      }
      frame 0 {
        w479 = u16 3 items=["总磷"=1, "氨氮"=3] ("站号")
        # "试剂填充 172 \n管路清洗108\n氨氮92\n总磷131\n总磷海水147\n总氮76\n总氮海水92"
        n256 = global read "VAR氨氮全局变量.vi" "状态告警区"() -> (w471:T10)
        n257 = Unbundle By Name(w471) -> ("系统时间"=w478:timestamp, "工作状态"=w469:T9)
        n258 = Bundle By Name(cluster=cluster{"命令":string, "data":variant} {"命令"="", "data"=variant} ("元素"), "命令"="读状态告警区", "data"=w479) -> (w482:cluster{"命令":string, "data":variant})
        n259 = Get Date/Time In Seconds() -> (seconds since 1Jan1904=w477:timestamp)
        n260 = Enqueue Element(queue=w470, element=w482) -> (queue out=w480:refnum<queue>)  [unwired: 2 in, 2 out]
        n261 = Subtract(x=w477, y=w478) -> (x-y=w476:dbl)
        n262 = Equal?(x=w469, y=T9."空闲") -> (x = y?=w467:bool)
        n263 = Absolute Value(x=w476) -> (abs(x)=w475:dbl)
        n264 = case shown="真" w467 {
          tunnel: w480 -> [w484 w487]
          tunnel: w479 -> [_ w486]
          tunnel: [w484 w485] -> w472
          frame False {
          }
          frame True {
            n265 = Bundle By Name(cluster=cluster{"命令":string, "data":variant} {"命令"="", "data"=variant} ("元素"), "命令"="读测量数据区", "data"=w486) -> (w489:cluster{"命令":string, "data":variant})
            n266 = Enqueue Element(queue=w487, element=w489) -> (queue out=w485:refnum<queue>)  [unwired: 2 in, 2 out]
          }
        }
        n267 = Greater Or Equal?(x=w475, y=120.0) -> (x >= y?=w473:bool)
        n268 = case shown="真" w473 {
          tunnel: w472 -> [_ w492]
          frame False {
          }
          frame True {
            n269 = call "氨氮启动命令.vi"("参数"=T29 {"站号"=3, "量程切换"=enum."AUTO", "控制命令"=enum."校时", "模式设置"=enum."待机", "测量间隔"=0}) -> ("启动命令"=w491:cluster{"命令":string, "data":variant})  [unwired: 10 in]
            n270 = Enqueue Element(queue=w492, element=w491) -> ()  [unwired: 2 in, 3 out]
          }
        }
      }
    }
    n271 = case shown="\"TCP\"" w461 {
      tunnel: [w494 w495] -> w462
      frame "串口", Default {
        n272 = global read "氨氮断电保存全局变量.vi" "VISA Resource"() -> (w494:refnum<visa-resource-name>)
      }
      frame "TCP" {
        n273 = global read "氨氮断电保存全局变量.vi" "IP"() -> (w495:string)
      }
    }
    "字符串" <- w462
    n274 = local write "流程路径"(w463) -> ()
    n275 = Wait (ms)(milliseconds to wait=u32 1000 ("等待时间（毫秒）")) -> ()  [unwired: 1 out]
  }
  n276 = control-ref of="公式"() -> (w21:refnum<vi>)
  n277 = control-ref of="量程参数读取"() -> (w11:refnum<vi>)
  n278 = control-ref of="参数下拉列表"() -> (w23:refnum<vi>)
  n279 = control-ref of="测量模式下拉列表"() -> (w22:refnum<vi>)
  n280 = control-ref of="量程下拉列表"() -> (w24:refnum<vi>)
  n281 = while {
    tunnel: w25 -> [w502]
    tunnel: w24 -> [w501]
    tunnel: w23 -> [w500]
    tunnel: w22 -> [w499]
    tunnel: w21 -> [w498]
    tunnel: w11 -> [w497]
    tunnel: w16 -> [_]
    tunnel: w12 -> [w496]
    stop <- FALSE stop-if-true
    n282 = event shown="[18] \"公式.X^2\", \"公式.X\", \"公式.b\", \"量程参数读取.测量精度\", \"量程参数读取.检出限\", \"量程参数读取.上限\", \"量程参数读取.下限\", \"量程参数读取.阈值（低->高）\", \"量程参数读取.阈值（高->低）\", \"量程参数读取.稀释度\": 鼠标按下" {
      selector: _ -> [_ _ _ _ _ _ _ _ _ _ _ _ _ _ _ _ _ _ _ _ _ _ _]
      dyn-events: _ -> [_ _ _ _ _ _ _ _ _ _ _ _ _ _ _ _ _ _ _ _ _ _ _]
      timeout: _ -> [_ _ _ _ _ _ _ _ _ _ _ _ _ _ _ _ _ _ _ _ _ _ _]
      tunnel: w502 -> [_ _ _ _ w522 w536 _ _ _ w554 _ _ _ w627 _ w640 _ _ _ _ _ _ _]
      tunnel: w501 -> [_ _ _ _ _ _ _ _ _ _ _ _ _ _ _ _ _ _ _ w656 _ _ _]
      tunnel: w500 -> [_ _ _ _ _ _ _ _ _ _ _ _ _ _ _ _ _ _ _ w654 _ w688 w695]
      tunnel: w499 -> [_ _ _ _ _ _ _ _ _ _ _ _ _ _ _ _ _ _ _ w655 _ _ _]
      tunnel: w498 -> [_ _ _ _ _ _ _ _ _ _ _ _ _ _ _ _ _ _ _ w652 _ _ _]
      tunnel: w497 -> [_ _ _ _ _ _ _ _ _ _ _ _ _ _ _ _ _ _ _ _ _ w686 _]
      tunnel: w496 -> [_ _ _ _ _ _ _ _ _ _ _ _ _ _ _ w635 _ _ _ _ _ _ _]
      tunnel: [_ _ _ w508 _ _ _ _ _ _ _ _ _ _ _ _ _ _ _ _ _ _ _] -> _
      event Timeout {
        n283 = event-data() -> ()  [unwired: 1 in, 3 out]
      }
      event "布尔": Mouse Down {
        n284 = event-data() -> ("CtlRef"=w505:refnum<vi>)  [unwired: 1 in, 5 out]
        n285 = property class="Bool (严格)"(reference=w505) -> ("Value"=w504:bool)  [unwired: 1 in, 2 out]
        n286 = case shown="真" w504 {
          frame False {
            n287 = call "密码键盘.vi"() -> ("NewNumber"=→"输入密码":dbl)  [unwired: 1 in]
          }
          frame True {
            n288 = local write "输入密码"(u32 0 ("输入密码")) -> ()
          }
        }
      }
      event "流程固件": Value Change {
        n289 = event-data() -> ()  [unwired: 1 in, 6 out]
        n290 = call "流程固件设置对话框.vi"() -> ()  [unwired: 12 in]
      }
      event "测量模式下拉列表", "量程下拉列表", "参数下拉列表": Value Change {
        n291 = event-data() -> ()  [unwired: 1 in, 6 out]
        n292 = local read "参数下拉列表"() -> (w510:enum16{"总磷", "总氮", "氨氮"})
        n293 = local read "测量模式下拉列表"() -> (w511:enum16{"水样测量", "零点核查", "跨度核查", "标样核查", "加标回收"})
        n294 = local read "量程下拉列表"() -> (w512:enum16{"低量程", "高量程"})
        n295 = Bundle("参数下拉列表"=w510, "测量模式下拉列表"=w511, "量程下拉列表"=w512) -> (w509:T28)  [unwired: 1 in]
        n296 = property on="曲线模型" class="曲线模型 (严格)"("属性"=w509) -> (error out=w508:errorcluster)  [unwired: 2 in, 1 out]
      }
      event "串口设置": Value Change {
        n297 = event-data() -> ()  [unwired: 1 in, 6 out]
        n298 = global read "氨氮断电保存全局变量.vi" "VISA Resource"() -> (w519:refnum<visa-resource-name>)
        n299 = global read "氨氮断电保存全局变量.vi" "MB通信方式选择"() -> (w513:enum16{"串口", "TCP"})
        n300 = global read "氨氮断电保存全局变量.vi" "IP"() -> (w518:string)
        n301 = global read "氨氮断电保存全局变量.vi" "PORT"() -> (w517:string)
        n302 = call "串口配置.vi"("PORT"=w517, "IP"=w518, "MB通信方式选择"=w513, "请选择串口:"=w519) -> ("PORT 2"=w515:string, "IP 2"=w516:string, "确认 2"=w520:bool, "VISA资源名称 2"=w521:refnum<visa-resource-name>, "MB通信方式选择 2"=w514:enum16{"串口", "TCP"})  [unwired: 3 in]
        n303 = case shown="真" w520 {
          tunnel: w521 -> [_ w527]
          tunnel: w522 -> [_ w526]
          tunnel: w516 -> [_ w525]
          tunnel: w515 -> [_ w524]
          tunnel: w514 -> [_ w523]
          frame False {
          }
          frame True {
            n304 = flat-sequence {
              tunnel: w527 -> [w532]
              tunnel: w526 -> [w533]
              tunnel: w525 -> [w531]
              tunnel: w524 -> [w530]
              tunnel: w523 -> [w529]
              frame #0 {
                n305 = global write "氨氮断电保存全局变量.vi" "VISA Resource"(w532) -> ()
                n306 = global write "氨氮断电保存全局变量.vi" "IP"(w531) -> ()
                n307 = global write "氨氮断电保存全局变量.vi" "PORT"(w530) -> ()
                n308 = global write "氨氮断电保存全局变量.vi" "MB通信方式选择"(w529) -> ()
                n309 = Flush Queue(queue=w533) -> (queue out=w528:refnum<queue>)  [unwired: 1 in, 2 out]
                n310 = Enqueue Element(queue=w528, element=cluster{"命令":string, "data":variant} {"命令"="启用模块", "data"=variant} ("元素")) -> ()  [unwired: 2 in, 3 out]
              }
              frame #1 {
                n311 = call "配置文件保存.vi"() -> ()  [unwired: 11 in, 1 out]
              }
            }
          }
        }
      }
      event "模块启用": Value Change {
        n312 = event-data() -> ("OldVal"=w537:bool)  [unwired: 1 in, 5 out]
        n313 = Flush Queue(queue=w536) -> (queue out=w535:refnum<queue>)  [unwired: 1 in, 2 out]
        n314 = case shown="假" w537 {
          tunnel: w535 -> [w538 w540]
          frame False {
            n315 = Enqueue Element(queue=w538, element=cluster{"命令":string, "data":variant} {"命令"="停用模块", "data"=variant} ("元素")) -> ()  [unwired: 2 in, 3 out]
          }
          frame True {
            n316 = Enqueue Element(queue=w540, element=cluster{"命令":string, "data":variant} {"命令"="启用模块", "data"=variant} ("元素")) -> ()  [unwired: 2 in, 3 out]
          }
        }
      }
      event "流程路径": Value Change {
        n317 = event-data() -> ()  [unwired: 1 in, 6 out]
        n318 = flat-sequence {
          frame #0 {
            n319 = local read "流程路径"() -> (w542:path)
            n320 = global write "氨氮断电保存全局变量.vi" "流程路径"(w542) -> ()
          }
          frame #1 {
            n321 = call "配置文件保存.vi"() -> ()  [unwired: 11 in, 1 out]
          }
        }
      }
      event "公式一键写入": Value Change {
        n322 = event-data() -> ()  [unwired: 1 in, 6 out]
        n323 = local read "公式"() -> (w543:cluster{"X^2":dbl, "X":dbl, "b":dbl})
        n324 = call "公式复合写入.vi"("公式"=w543) -> ()  [unwired: 11 in]
      }
      event "曲线模型": Value Change {
        n325 = event-data() -> ()  [unwired: 1 in, 6 out]
        n326 = Unbundle By Name("曲线模型") -> ("X^2"=w546:dbl, "X"=w547:dbl, "B"=w548:dbl)
        n327 = Build Array(w546, w547, w548) -> (w545:dbl[])
        n328 = Array To Cluster(array=w545) -> (cluster=w544:cluster{"[0]":dbl, "[1]":dbl, "[2]":dbl})
        n329 = local write "公式"(w544) -> ()
      }
      event "校准按钮.校准1", "校准按钮.校准2", "校准按钮.校准3", "校准按钮.校准4", "校准按钮.校准5": Value Change {
        n330 = event-data() -> ("CtlRef"=w561:refnum<vi>)  [unwired: 1 in, 5 out]
        n331 = property class="Bool"(reference=w561) -> ("Label.Text"=w560:string)  [unwired: 1 in, 2 out]
        n332 = property on="曲线模型" class="曲线模型 (严格)"() -> ("浓度属性"=w557:T30)  [unwired: 2 in, 2 out]
        n333 = case shown="\"校准3\"" w560 {
          tunnel: [w567 w570 w573 w576 w579] -> w553
          tunnel: [u16 1 ("校准点1-5") u16 2 ("校准点1-5") u16 3 ("校准点1-5") u16 4 ("校准点1-5") u16 5 ("校准点1-5")] -> w558
          tunnel: w557 -> [w568 w571 w574 w577 w580]
          frame "校准1", Default {
            n334 = Unbundle By Name(w568) -> ("标液浓度1"=w567:dbl)
          }
          frame "校准2" {
            n335 = Unbundle By Name(w571) -> ("标液浓度2"=w570:dbl)
          }
          frame "校准3" {
            n336 = Unbundle By Name(w574) -> ("标液浓度3"=w573:dbl)
          }
          frame "校准4" {
            n337 = Unbundle By Name(w577) -> ("标液浓度4"=w576:dbl)
          }
          frame "校准5" {
            n338 = Unbundle By Name(w580) -> ("标液浓度5"=w579:dbl)
          }
        }
        n339 = Not Equal To 0?(x=w553) -> (x != 0?=w552:bool)
        n340 = Bundle By Name(cluster=cluster{"校准？":bool, "校准点1-5":u16, "校准浓度":dbl} {"校准？"=FALSE, "校准点1-5"=0, "校准浓度"=0.0} ("校准输出"), "校准？"=TRUE, "校准点1-5"=w558, "校准浓度"=w553) -> (w556:cluster{"校准？":bool, "校准点1-5":u16, "校准浓度":dbl})
        n341 = global write "氨氮断电保存全局变量.vi" "校准输出"(w556) -> ()
        n342 = local read "量程下拉列表"() -> (w550:enum16{"低量程", "高量程"})
        n343 = case shown="假" w552 {
          tunnel: [cluster{"命令":string, "data":variant} {"命令"="启动", "data"=variant(cluster{"站号":u16, "控制命令":u16[]} {"站号"=3, "控制命令"=[2048, 256]})} ("元素") w564] -> w551
          tunnel: w550 -> [_ w563]
          frame False {
            # "校零"
          }
          frame True {
            # "校标"
            n344 = case shown="\"高量程\"" w563 {
              tunnel: [cluster{"命令":string, "data":variant} {"命令"="启动", "data"=variant(cluster{"站号":u16, "控制命令":u16[]} {"站号"=3, "控制命令"=[2304, 256]})} ("元素") cluster{"命令":string, "data":variant} {"命令"="启动", "data"=variant(cluster{"站号":u16, "控制命令":u16[]} {"站号"=3, "控制命令"=[2304, 257]})} ("元素")] -> w564
              frame "低量程", Default {
              }
              frame "高量程" {
              }
            }
          }
        }
        n345 = Enqueue Element(queue=w554, element=w551) -> ()  [unwired: 2 in, 3 out]
      }
      event "质控参数设置": Value Change {
        n346 = event-data() -> ()  [unwired: 1 in, 6 out]
        n347 = global read "氨氮断电保存全局变量.vi" "质控参数设置"() -> (w582:T31)
        n348 = call "质控参数设置.vi"("质控参数设置"=w582) -> ("输出簇"=w583:T32)  [unwired: 10 in]
        n349 = Unbundle By Name(w583) -> ("确定"=w584:bool)
        n350 = case shown="真" w584 {
          tunnel: w583 -> [_ w586]
          tunnel: w582 -> [_ w585]
          frame False {
          }
          frame True {
            n351 = flat-sequence {
              tunnel: w586 -> [w593]
              tunnel: w585 -> [w592]
              frame #0 {
                n352 = Unbundle By Name(w593) -> ("跨度值"=w591:dbl, "零点标准液浓度"=w590:dbl, "跨度标准液浓度"=w589:dbl, "标准液标准浓度"=w588:dbl)
                n353 = Bundle By Name(cluster=w592, "跨度值"=w591, "零点标准液浓度"=w590, "跨度标准液浓度"=w589, "标准液标准浓度"=w588) -> (w587:T31)
                n354 = global write "氨氮断电保存全局变量.vi" "质控参数设置"(w587) -> ()
              }
              frame #1 {
                n355 = call "配置文件保存.vi"() -> ()  [unwired: 11 in, 1 out]
              }
            }
          }
        }
      }
      event "仪器参数设置": Value Change {
        n356 = event-data() -> ()  [unwired: 1 in, 6 out]
        n357 = global read "氨氮断电保存全局变量.vi" "氨氮仪器参数"() -> (w594:T33)
        n358 = call "仪器参数设置.vi"("氨氮仪器参数"=w594) -> ("仪器参数设置输出"=w595:T34)  [unwired: 10 in]
        n359 = Unbundle By Name(w595) -> ("确定"=w596:bool)
        n360 = case shown="真" w596 {
          tunnel: w595 -> [_ w598]
          tunnel: w594 -> [_ w597]
          frame False {
          }
          frame True {
            n361 = flat-sequence {
              tunnel: w598 -> [w614]
              tunnel: w597 -> [w613]
              frame #0 {
                n362 = Unbundle By Name(w614) -> ("测量量程"=w612:dbl, "测量精度"=w611:dbl, "测量间隔"=w610:dbl, "消解温度"=w609:dbl, "消解时长"=w607:dbl, "空白校准时间"=w606:timestamp, "曲线截距"=w605:dbl, "曲线斜率"=w604:dbl, "测量检出限"=w603:dbl, "测量信号值"=w602:dbl, "线性相关系数"=w601:dbl, "二次多项式系数"=w600:dbl, "标样校准时间"=w599:timestamp)
                n363 = Bundle By Name(cluster=w613, "测量量程"=w612, "测量精度"=w611, "测量间隔"=w610, "消解温度"=w609, "消解时长"=w607, "空白校准时间"=w606, "曲线截距"=w605, "曲线斜率"=w604, "测量检出限"=w603, "测量信号值"=w602, "线性相关系数"=w601, "二次多项式系数"=w600, "标样校准时间"=w599) -> (w608:T33)
                n364 = global write "氨氮断电保存全局变量.vi" "氨氮仪器参数"(w608) -> ()
              }
              frame #1 {
                n365 = call "配置文件保存.vi"() -> ()  [unwired: 11 in, 1 out]
              }
            }
          }
        }
      }
      event "自动测试量程配置": Value Change {
        n366 = event-data() -> ()  [unwired: 1 in, 6 out]
        n367 = flat-sequence {
          frame #0 {
            n368 = global write "氨氮断电保存全局变量.vi" "自动测试量程配置"("自动测试量程配置") -> ()
          }
          frame #1 {
            n369 = call "配置文件保存.vi"() -> ()  [unwired: 11 in, 1 out]
          }
        }
      }
      event "手动启动": Value Change {
        n370 = event-data() -> ()  [unwired: 1 in, 6 out]
        n371 = call "氨氮启动参数对话框.vi"() -> ("标样浓度输出"=w616:dbl, "确认"=w626:bool, "元素"=w625:cluster{"命令":string, "data":variant})  [unwired: 9 in]
        n372 = case shown="真" w626 {
          tunnel: w627 -> [_ w633]
          tunnel: w625 -> [_ w632]
          frame False {
          }
          frame True {
            n373 = Enqueue Element(queue=w633, element=w632) -> ()  [unwired: 2 in, 3 out]
          }
        }
        n374 = Unbundle By Name(w625) -> ("data"=w623:variant)
        n375 = Variant To Data(type=cluster{"站号":u16, "控制命令":u16[]} {"站号"=0, "控制命令"=[]} ("输出簇"), Variant=w623) -> (data=w622:cluster{"站号":u16, "控制命令":u16[]})  [unwired: 1 in, 1 out]
        n376 = Unbundle By Name(w622) -> ("控制命令"=w621:u16[])
        n377 = Index Array(array=w621) -> (element=w620:u16)  [unwired: 1 in]
        n378 = Swap Bytes(anything=w620) -> (byte swapped=w619:u16)
        n379 = Equal?(x=w619, y=u16 2) -> (x = y?=w617:bool)
        n380 = case shown="真" w617 {
          tunnel: w616 -> [_ w628]
          frame False {
          }
          frame True {
            n381 = flat-sequence {
              tunnel: w628 -> [w629]
              frame #0 {
                n382 = global read "氨氮断电保存全局变量.vi" "质控参数设置"() -> (w631:T31)
                n383 = Bundle By Name(cluster=w631, "标准液标准浓度"=w629) -> (w630:T31)
                n384 = global write "氨氮断电保存全局变量.vi" "质控参数设置"(w630) -> ()
              }
              frame #1 {
                n385 = call "配置文件保存.vi"() -> ()  [unwired: 11 in, 1 out]
              }
            }
          }
        }
      }
      event "单步测试": Value Change {
        n386 = event-data() -> ()  [unwired: 1 in, 6 out]
        n387 = call "氨氮单步调试对话框.vi"() -> ()  [unwired: 12 in]
      }
      event "停止": Value Change {
        n388 = event-data() -> ()  [unwired: 1 in, 6 out]
        n389 = Cancel Notification(0:w635) -> (8:w636:refnum<notifier>)  [unwired: 1 in, 2 out]
        n390 = Enqueue Element(queue=w640, element=cluster{"命令":string, "data":variant} {"命令"="启动", "data"=variant(cluster{"站号":u16, "控制命令输出":u16[]} {"站号"=1, "控制命令输出"=[2816]})} ("元素")) -> (queue out=w637:refnum<queue>)  [unwired: 2 in, 2 out]
        n391 = Send Notification(notification=TRUE ("通知"), notifier=w636) -> ()  [unwired: 1 in, 2 out]
        n392 = Enqueue Element(queue=w637, element=cluster{"命令":string, "data":variant} {"命令"="启动", "data"=variant(cluster{"站号":u16, "控制命令输出":u16[]} {"站号"=2, "控制命令输出"=[2816]})} ("元素")) -> ()  [unwired: 2 in, 3 out]
      }
      event "设置": Value Change {
        n393 = event-data() -> ()  [unwired: 1 in, 6 out]
        n394 = property on="窗格" class="Pane"("Origin"=T18 {"Horizontal"=0, "Vertical"=628} ("原点")) -> ()  [unwired: 2 in, 2 out]
      }
      event "返回": Value Change {
        n395 = event-data() -> ()  [unwired: 1 in, 6 out]
        n396 = property on="窗格" class="Pane"("Origin"=T18 {"Horizontal"=0, "Vertical"=0} ("原点")) -> ()  [unwired: 2 in, 2 out]
      }
      event "公式.X^2", "公式.X", "公式.b", "量程参数读取.测量精度", "量程参数读取.检出限", "量程参数读取.上限", "量程参数读取.下限", "量程参数读取.阈值（低->高）", "量程参数读取.阈值（高->低）", "量程参数读取.稀释度": Mouse Down {
        n397 = event-data() -> ("CtlRef"=w646:refnum<vi>)  [unwired: 1 in, 5 out]
        n398 = property class="DigNum (严格)"(reference=w646) -> (reference out=w644:refnum<vi>, "Value"=w645:dbl)  [unwired: 1 in, 1 out]
        n399 = call "数字键盘.vi"("OldNumber"=w645) -> ("NewNumber"=w643:dbl)
        n400 = property class="DigNum (严格)"(reference=w644, "Val(Sgnl)"=w643) -> ()  [unwired: 1 in, 2 out]
      }
      event "读公式": Value Change {
        n401 = event-data() -> ()  [unwired: 1 in, 6 out]
        n402 = property class="Enum (严格)"(reference=w654) -> ("Value"=w653:enum16{"总磷", "总氮", "氨氮"})  [unwired: 1 in, 2 out]
        n403 = property class="Enum (严格)"(reference=w655) -> ("Value"=w650:enum16{"水样测量", "零点核查", "跨度核查", "标样核查", "加标回收"})  [unwired: 1 in, 2 out]
        n404 = property class="Enum (严格)"(reference=w656) -> ("Value"=w649:enum16{"低量程", "高量程"})  [unwired: 1 in, 2 out]
        n405 = call "公式读取.vi"("量程"=w649, "测量模式"=w650, "测量参数"=w653) -> ("error out"=w647:errorcluster, "公式"=w648:cluster{"X^2":dbl, "X":dbl, "b":dbl})  [unwired: 7 in]
        n406 = property class="Clust (严格)"(reference=w652, "Value"=w648) -> ()  [unwired: 1 in, 2 out]
        n407 = case shown="无错误" w647 {
          tunnel: ["读取成功" ("消息") "读取失败" ("消息")] -> w651
          frame No Error {
          }
          frame Error {
          }
        }
        n408 = One Button Dialog(message=w651) -> ()  [unwired: 1 in, 1 out]
      }
      event "写公式": Value Change {
        n409 = event-data() -> ()  [unwired: 1 in, 6 out]
        n410 = call "公式写入.vi"("公式"="公式", "量程"="量程下拉列表", "测量模式"="测量模式下拉列表", "测量参数"="参数下拉列表") -> ("error out"=w663:errorcluster)  [unwired: 7 in]
        n411 = case shown="无错误" w663 {
          tunnel: ["写入成功" ("消息") "写入失败" ("消息")] -> w664
          tunnel: "测量模式下拉列表" -> [w673 _]
          tunnel: "量程下拉列表" -> [w672 _]
          tunnel: "公式" -> [w668 _]
          frame No Error {
            n412 = Unbundle By Name(w668) -> ("X^2"=w667:dbl, "X"=w666:dbl, "b"=w665:dbl)
            n413 = Equal?(x=w673, y=enum16{"水样测量", "零点核查", "跨度核查", "标样核查", "加标回收"}."水样测量") -> (x = y?=w671:bool)
            n414 = Equal?(x=w672, y=enum16{"低量程", "高量程"}."低量程") -> (x = y?=w670:bool)
            n415 = Compound Arithmetic op=AND ("复合运算")(w671, w670) -> (w669:bool)
            n416 = case shown="真" w669 {
              tunnel: w667 -> [_ w679]
              tunnel: w666 -> [_ w678]
              tunnel: w665 -> [_ w677]
              frame False {
              }
              frame True {
                n417 = global read "氨氮断电保存全局变量.vi" "氨氮仪器参数"() -> (w680:T33)
                n418 = Bundle By Name(cluster=w680, "曲线截距"=w677, "曲线斜率"=w678, "二次多项式系数"=w679) -> (w681:T33)
                n419 = global write "氨氮断电保存全局变量.vi" "氨氮仪器参数"(w681) -> ()
              }
            }
          }
          frame Error {
          }
        }
        n420 = One Button Dialog(message=w664) -> ()  [unwired: 1 in, 1 out]
      }
      event "量程切换阈值读取": Value Change {
        n421 = event-data() -> ()  [unwired: 1 in, 6 out]
        n422 = property class="Enum (严格)"(reference=w688) -> ("Value"=w687:enum16{"总磷", "总氮", "氨氮"})  [unwired: 1 in, 2 out]
        n423 = call "量程读取.vi"("测量参数"=w687) -> ("error out"=w683:errorcluster, "量程参数读取"=w685:T35)  [unwired: 9 in]
        n424 = property class="Clust (严格)"(reference=w686, "Value"=w685) -> ()  [unwired: 1 in, 2 out]
        n425 = case shown="错误" w683 {
          tunnel: ["读取成功" ("消息") "读取失败" ("消息")] -> w684
          frame No Error {
          }
          frame Error {
          }
        }
        n426 = One Button Dialog(message=w684) -> ()  [unwired: 1 in, 1 out]
      }
      event "量程切换阈值写入": Value Change {
        n427 = event-data() -> ()  [unwired: 1 in, 6 out]
        n428 = property class="Enum (严格)"(reference=w695) -> ("Value"=w694:enum16{"总磷", "总氮", "氨氮"})  [unwired: 1 in, 2 out]
        n429 = call "量程写入.vi"("量程参数写入"="量程参数读取", "测量参数"=w694) -> ("error out"=w692:errorcluster)  [unwired: 8 in]
        n430 = case shown="无错误" w692 {
          tunnel: ["写入成功" ("消息") "写入失败" ("消息")] -> w693
          frame No Error {
          }
          frame Error {
          }
        }
        n431 = One Button Dialog(message=w693) -> ()  [unwired: 1 in, 1 out]
      }
    }
  }
  n432 = while {
    tunnel: [w705] -> _
    shift-right: [w703] -> _
    shift-left: w4 -> [w702]
    tunnel: w5 -> [w699]
    stop <- FALSE stop-if-true
    n433 = global read "VAR氨氮全局变量.vi" "配置文件 path"() -> (w698:path)
    n434 = Read from Text File(file (use dialog)=w698, error in=w699) -> (text=w703:string, error out=w700:errorcluster)  [unwired: 2 in, 2 out]
    n435 = Not Equal?(x=w703, y=w702) -> (x != y?=w701:bool)
    n436 = case shown="真" w701 {
      tunnel: [w707 w711] -> w705
      tunnel: w698 -> [_ w710]
      tunnel: w700 -> [w707 w709]
      frame False {
      }
      frame True {
        # "文件发生改变进行更新"
        n437 = call <vilib>:"Open Config Data.vi"("error in (no error)"=w709, "configuration file path"=w710) -> ("error out"=w715:errorcluster, "refnum"=w714:T21)  [unwired: 7 in, 1 out]
        n438 = vi-ref "氨氮断电保存全局变量.vi"() -> (w708:refnum<vi>)
        n439 = call <userlib>:"Read Panel from INI__ogtk.vi"("error in (no error)"=w715, "VI ref"=w708, "refnum"=w714) -> ("error out"=w713:errorcluster, "refnum out"=w712:T21)  [unwired: 7 in]
        n440 = call <vilib>:"Close Config Data.vi"("error in (no error)"=w713, "refnum"=w712) -> ("error out"=w711:errorcluster)  [unwired: 8 in, 1 out]
      }
    }
    n441 = Wait (ms)(milliseconds to wait=u32 1000 ("等待时间（毫秒）")) -> ()  [unwired: 1 out]
  }
